vi "test.OutputStream.vi"(8 "error in":errorcluster, 10 "Data":variant, 11 "Command":string) -> (0 "error out":errorcluster, 3 "Return Data":variant)   [LabVIEW 2014]
uses:
  Private/Class/meth.Constructor.vi
  Private/Class/meth.SetStreamReader.vi
  Private/Class/meth.Destructor.vi
  Private/Class/meth.ExecFunction.vi
  GLue.lvlib
panel:
  out "String":string
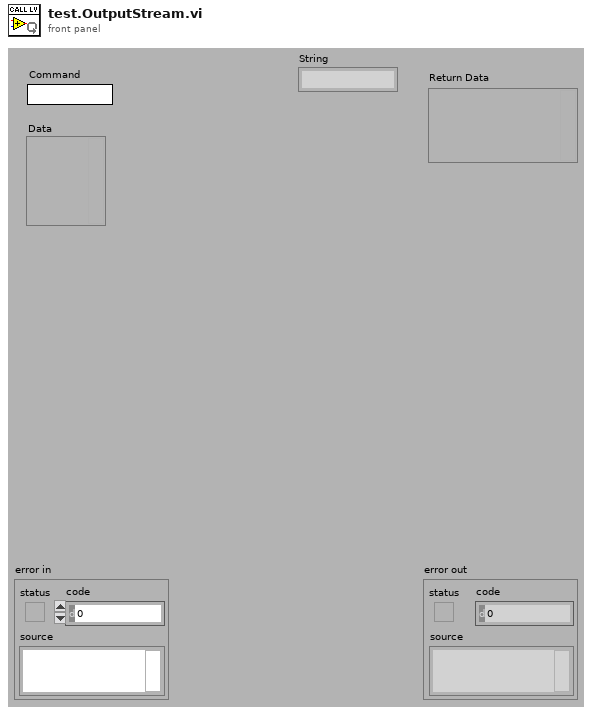
[diagram p1: front panel]
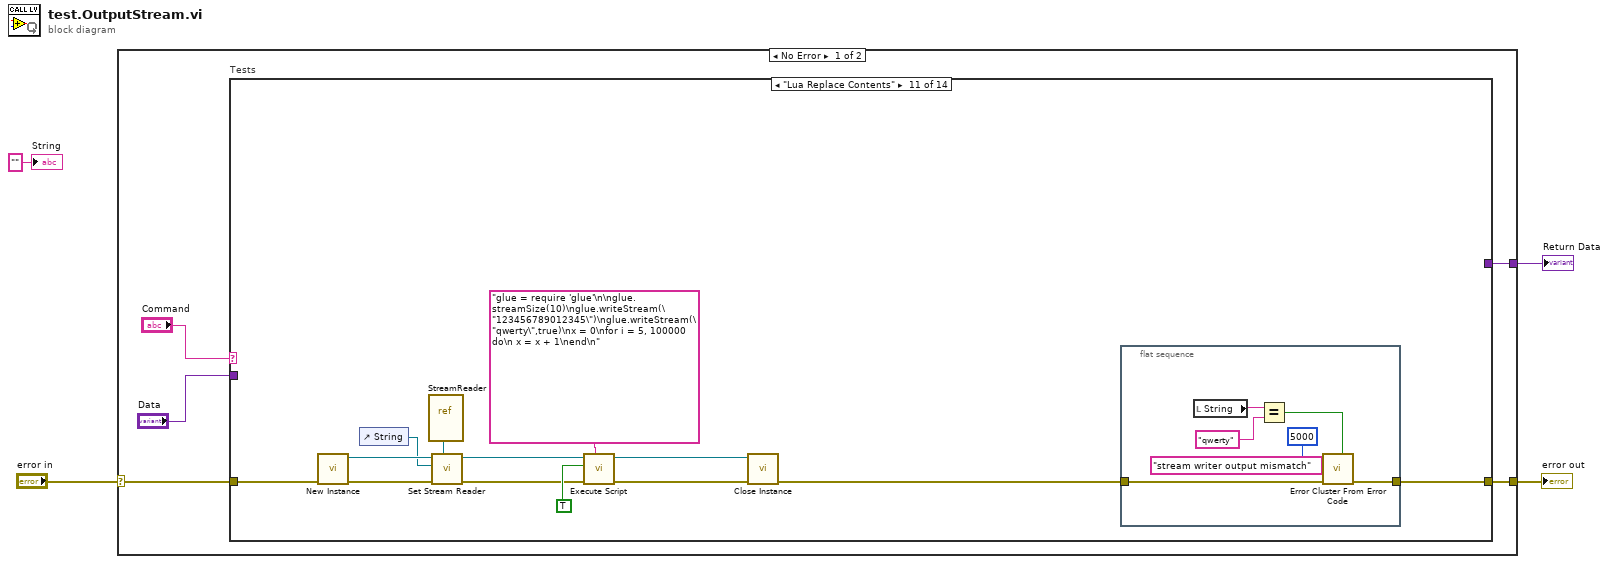
[diagram p0: block diagram]
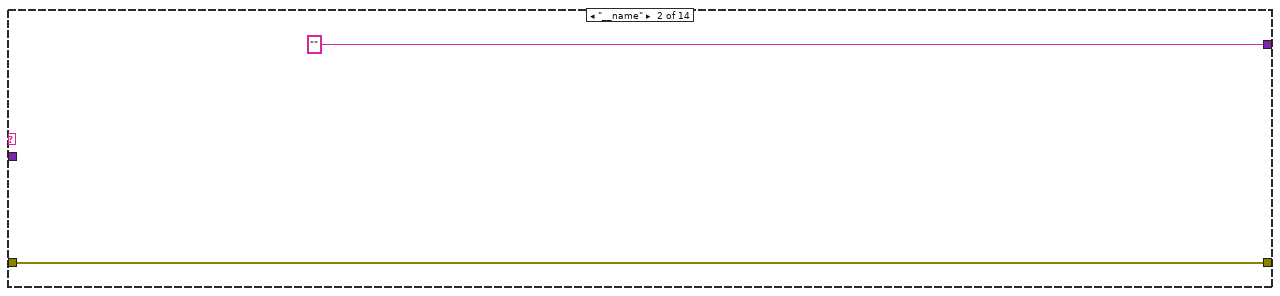
[diagram p3: hidden frame]
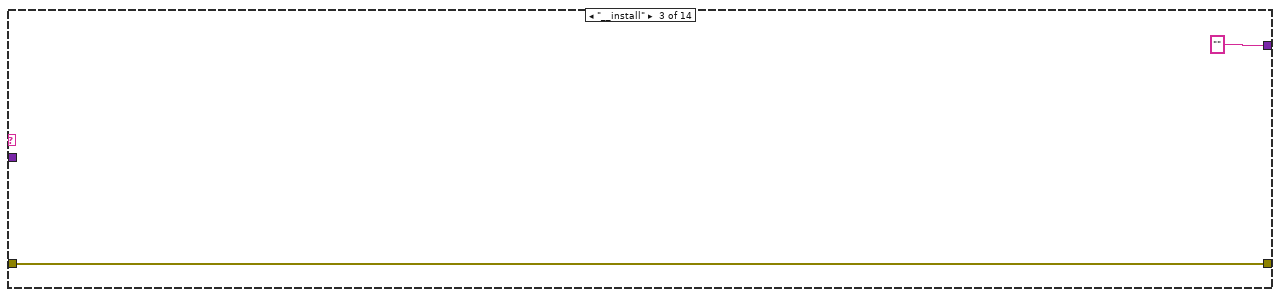
[diagram p4: hidden frame]
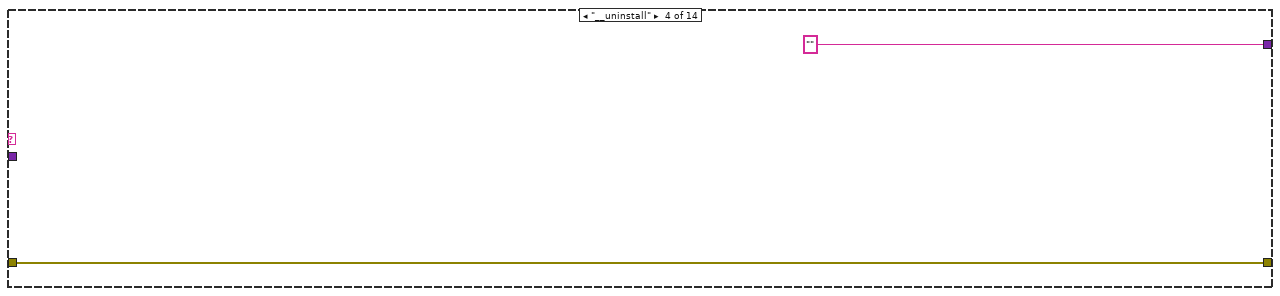
[diagram p5: hidden frame]
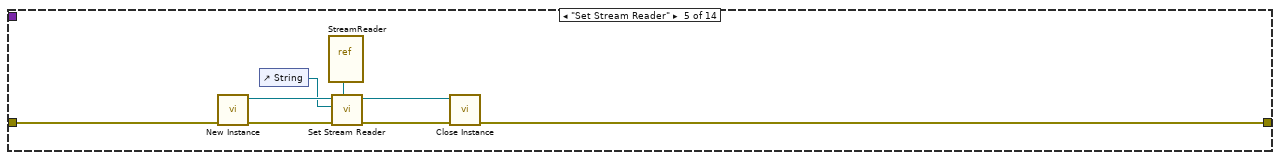
[diagram p6: hidden frame]
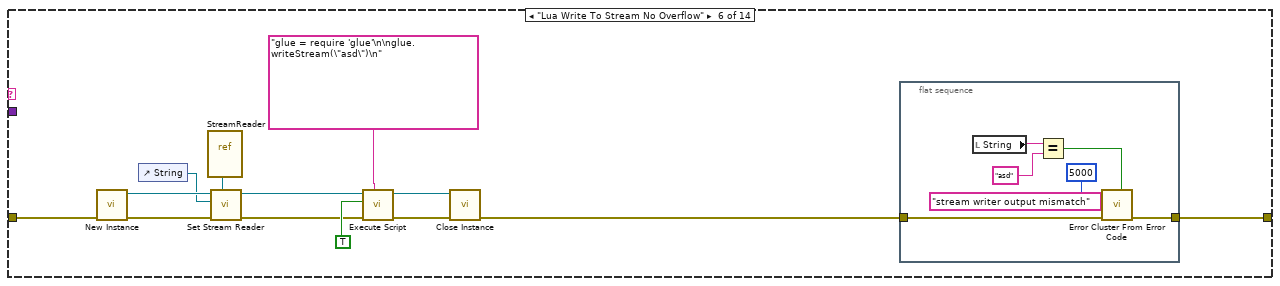
[diagram p7: hidden frame]
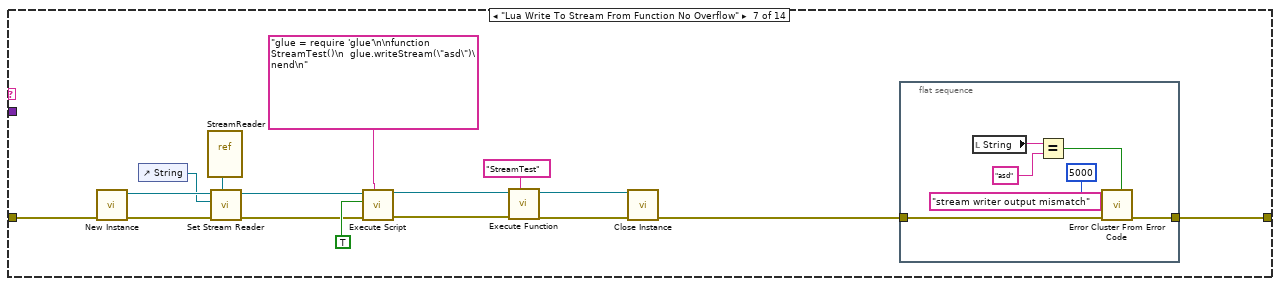
[diagram p8: hidden frame]
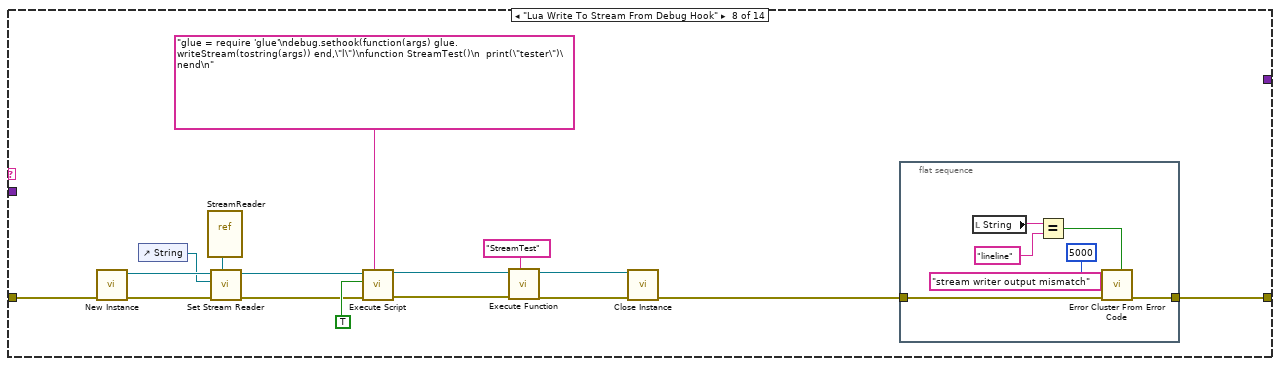
[diagram p9: hidden frame]
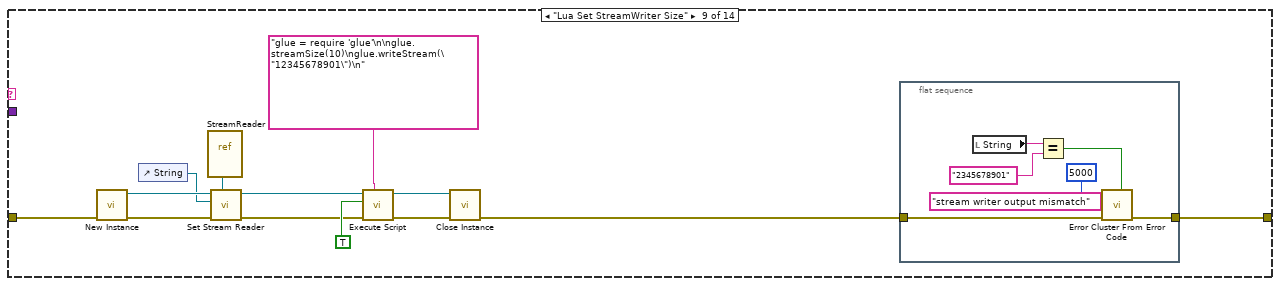
[diagram p10: hidden frame]
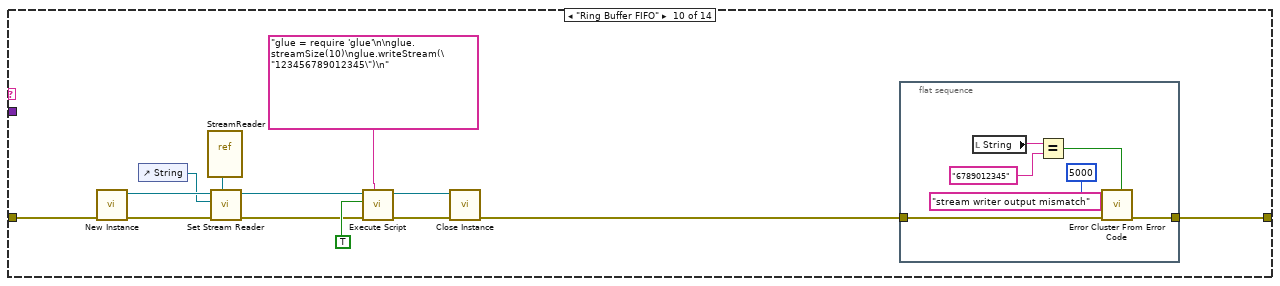
[diagram p11: hidden frame]
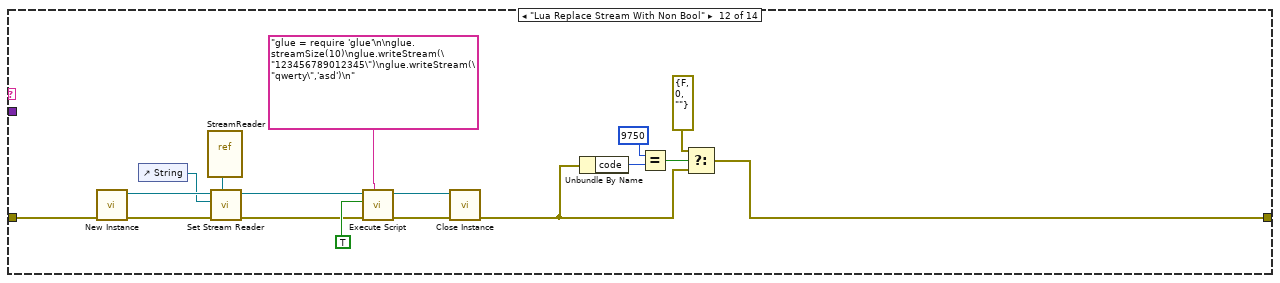
[diagram p12: hidden frame]
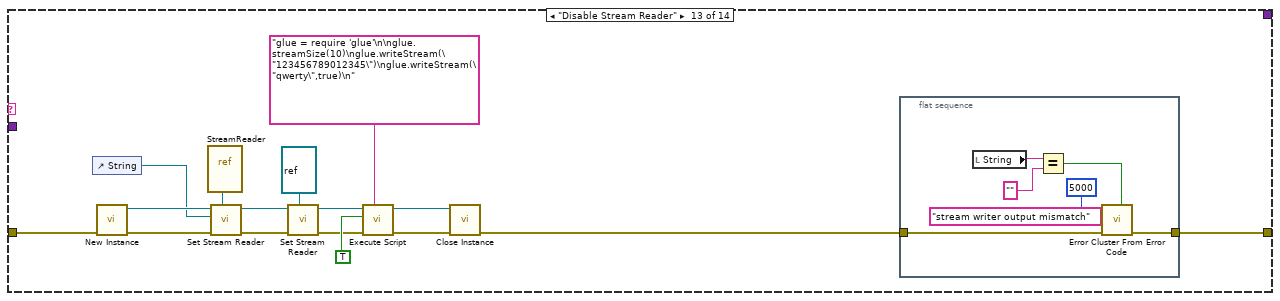
[diagram p13: hidden frame]
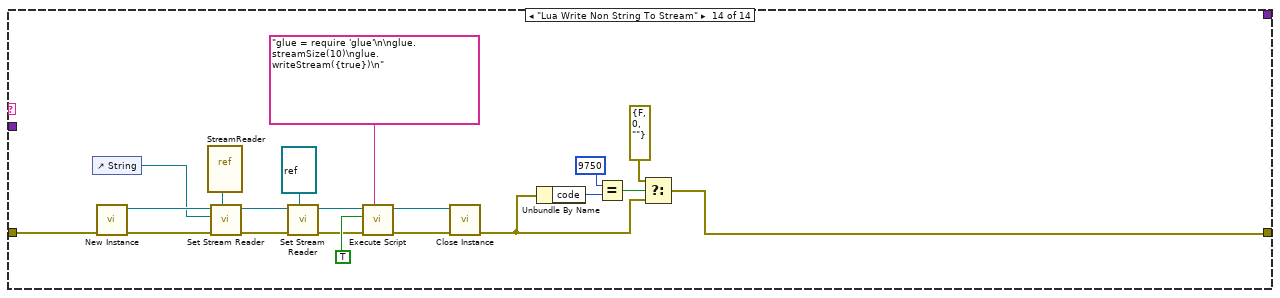
[diagram p14: hidden frame]
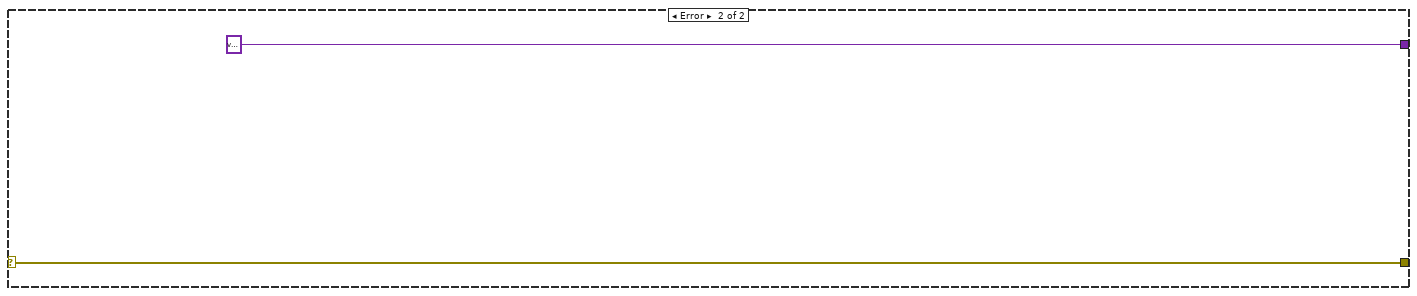
[diagram p15: hidden frame]
diagram:
  n1 = case shown="No Error" "error in" {
    selector: "error in" -> [w9 w213]
    tunnel: [w7 w213] -> w3
    tunnel: [w8 variant ("User Data")] -> w2
    frame No Error {
      n2 = case "Tests" shown="\"Lua Replace Contents\"" "Command" {
        tunnel: w9 -> [w11 w12 w14 w16 w25 w38 w61 w84 w104 w124 w144 w168 w184 w211]
        tunnel: "Data" -> [w10 _ _ _ _ _ _ _ _ _ _ _ _ _]
        tunnel: [w10 "" "" "" _ _ _ _ _ _ _ _ _ _] -> w8
        tunnel: [w11 w12 w14 w16 w24 w26 w51 w74 w92 w112 w132 w152 w174 w192] -> w7
        frame Default {
        }
        frame "__name" {
        }
        frame "__install" {
        }
        frame "__uninstall" {
        }
        frame "Set Stream Reader" {
          n3 = call "New Instance.vi"("error in"=w25) -> ("error out"=w23:errorcluster, "GLue out"=w22:refnum<class "class.GLue.lvclass">)  [unwired: 9 in]
          n4 = control-ref of="String"() -> (w20:refnum<vi>)
          n5 = vi-ref "StreamReader.vi"() -> (w21:refnum<vi>)
          n6 = call "Set Stream Reader.vi"("StreamReader"=w21, "error in"=w23, "UserData"=w20, "GLue in"=w22) -> ("error out"=w19:errorcluster, "GLue out"=w18:refnum<class "class.GLue.lvclass">)  [unwired: 6 in]
          n7 = call "Close Instance.vi"("error in"=w19, "GLue in"=w18) -> ("error out"=w24:errorcluster)  [unwired: 9 in]
        }
        frame "Lua Write To Stream No Overflow" {
          n8 = call "New Instance.vi"("error in"=w38) -> ("error out"=w33:errorcluster, "GLue out"=w30:refnum<class "class.GLue.lvclass">)  [unwired: 9 in]
          n9 = control-ref of="String"() -> (w28:refnum<vi>)
          n10 = vi-ref "StreamReader.vi"() -> (w29:refnum<vi>)
          n11 = call "Set Stream Reader.vi"("StreamReader"=w29, "error in"=w33, "UserData"=w28, "GLue in"=w30) -> ("error out"=w32:errorcluster, "GLue out"=w31:refnum<class "class.GLue.lvclass">)  [unwired: 6 in]
          n12 = call "Execute Script.vi"("Script"="glue = require 'glue'\n\nglue.writeStream(\"asd\")\n", "error in"=w32, "Argument Data"=TRUE, "GLue in"=w31) -> ("error out"=w35:errorcluster, "GLue out"=w34:refnum<class "class.GLue.lvclass">)  [unwired: 5 in, 1 out]
          n13 = call "Close Instance.vi"("error in"=w35, "GLue in"=w34) -> ("error out"=w27:errorcluster)  [unwired: 9 in]
          n14 = flat-sequence {
            tunnel: w27 -> [w43]
            tunnel: [w42] -> w26
            frame #0 {
              n15 = local read "String"() -> (w45:string)
              n16 = Equal?(x=w45, y="asd") -> (x = y?=w41:bool)
              n17 = call <vilib>:"Error Cluster From Error Code.vi"("is warning? (False)"=w41, "error in (no error)"=w43, "error message (\"\")"="stream writer output mismatch" ("error message (\"\")"), "error code (0)"=5000) -> ("error out"=w42:errorcluster)  [unwired: 5 in]
            }
          }
        }
        frame "Lua Write To Stream From Function No Overflow" {
          n18 = call "New Instance.vi"("error in"=w61) -> ("error out"=w58:errorcluster, "GLue out"=w55:refnum<class "class.GLue.lvclass">)  [unwired: 9 in]
          n19 = control-ref of="String"() -> (w53:refnum<vi>)
          n20 = vi-ref "StreamReader.vi"() -> (w54:refnum<vi>)
          n21 = call "Set Stream Reader.vi"("StreamReader"=w54, "error in"=w58, "UserData"=w53, "GLue in"=w55) -> ("error out"=w57:errorcluster, "GLue out"=w56:refnum<class "class.GLue.lvclass">)  [unwired: 6 in]
          n22 = call "Execute Script.vi"("Script"="glue = require 'glue'\n\nfunction StreamTest()\n  glue.writeStream(\"asd\")\nend\n", "error in"=w57, "Argument Data"=TRUE, "GLue in"=w56) -> ("error out"=w50:errorcluster, "GLue out"=w49:refnum<class "class.GLue.lvclass">)  [unwired: 5 in, 1 out]
          n23 = call "Execute Function.vi"("Function Name"="StreamTest", "error in"=w50, "GLue in"=w49) -> ("error out"=w47:errorcluster, "GLue out"=w48:refnum<class "class.GLue.lvclass">)  [unwired: 6 in, 1 out]
          n24 = call "Close Instance.vi"("error in"=w47, "GLue in"=w48) -> ("error out"=w52:errorcluster)  [unwired: 9 in]
          n25 = flat-sequence {
            tunnel: w52 -> [w66]
            tunnel: [w65] -> w51
            frame #0 {
              n26 = local read "String"() -> (w68:string)
              n27 = Equal?(x=w68, y="asd") -> (x = y?=w64:bool)
              n28 = call <vilib>:"Error Cluster From Error Code.vi"("is warning? (False)"=w64, "error in (no error)"=w66, "error message (\"\")"="stream writer output mismatch" ("error message (\"\")"), "error code (0)"=5000) -> ("error out"=w65:errorcluster)  [unwired: 5 in]
            }
          }
        }
        frame "Lua Write To Stream From Debug Hook" {
          n29 = call "New Instance.vi"("error in"=w84) -> ("error out"=w81:errorcluster, "GLue out"=w78:refnum<class "class.GLue.lvclass">)  [unwired: 9 in]
          n30 = control-ref of="String"() -> (w76:refnum<vi>)
          n31 = vi-ref "StreamReader.vi"() -> (w77:refnum<vi>)
          n32 = call "Set Stream Reader.vi"("StreamReader"=w77, "error in"=w81, "UserData"=w76, "GLue in"=w78) -> ("error out"=w80:errorcluster, "GLue out"=w79:refnum<class "class.GLue.lvclass">)  [unwired: 6 in]
          n33 = call "Execute Script.vi"("Script"="glue = require 'glue'\ndebug.sethook(function(args) glue.writeStream(tostring(args)) end,\"l\")\nfunction StreamTest()\n  print(\"tester\")\nend\n", "error in"=w80, "Argument Data"=TRUE, "GLue in"=w79) -> ("error out"=w73:errorcluster, "GLue out"=w72:refnum<class "class.GLue.lvclass">)  [unwired: 5 in, 1 out]
          n34 = call "Execute Function.vi"("Function Name"="StreamTest", "error in"=w73, "GLue in"=w72) -> ("error out"=w70:errorcluster, "GLue out"=w71:refnum<class "class.GLue.lvclass">)  [unwired: 6 in, 1 out]
          n35 = call "Close Instance.vi"("error in"=w70, "GLue in"=w71) -> ("error out"=w75:errorcluster)  [unwired: 9 in]
          n36 = flat-sequence {
            tunnel: w75 -> [w89]
            tunnel: [w88] -> w74
            frame #0 {
              n37 = local read "String"() -> (w91:string)
              n38 = Equal?(x=w91, y="lineline") -> (x = y?=w87:bool)
              n39 = call <vilib>:"Error Cluster From Error Code.vi"("is warning? (False)"=w87, "error in (no error)"=w89, "error message (\"\")"="stream writer output mismatch" ("error message (\"\")"), "error code (0)"=5000) -> ("error out"=w88:errorcluster)  [unwired: 5 in]
            }
          }
        }
        frame "Lua Set StreamWriter Size" {
          n40 = call "New Instance.vi"("error in"=w104) -> ("error out"=w99:errorcluster, "GLue out"=w96:refnum<class "class.GLue.lvclass">)  [unwired: 9 in]
          n41 = control-ref of="String"() -> (w94:refnum<vi>)
          n42 = vi-ref "StreamReader.vi"() -> (w95:refnum<vi>)
          n43 = call "Set Stream Reader.vi"("StreamReader"=w95, "error in"=w99, "UserData"=w94, "GLue in"=w96) -> ("error out"=w98:errorcluster, "GLue out"=w97:refnum<class "class.GLue.lvclass">)  [unwired: 6 in]
          n44 = call "Execute Script.vi"("Script"="glue = require 'glue'\n\nglue.streamSize(10)\nglue.writeStream(\"12345678901\")\n", "error in"=w98, "Argument Data"=TRUE, "GLue in"=w97) -> ("error out"=w101:errorcluster, "GLue out"=w100:refnum<class "class.GLue.lvclass">)  [unwired: 5 in, 1 out]
          n45 = call "Close Instance.vi"("error in"=w101, "GLue in"=w100) -> ("error out"=w93:errorcluster)  [unwired: 9 in]
          n46 = flat-sequence {
            tunnel: w93 -> [w109]
            tunnel: [w108] -> w92
            frame #0 {
              n47 = local read "String"() -> (w111:string)
              n48 = Equal?(x=w111, y="2345678901") -> (x = y?=w107:bool)
              n49 = call <vilib>:"Error Cluster From Error Code.vi"("is warning? (False)"=w107, "error in (no error)"=w109, "error message (\"\")"="stream writer output mismatch" ("error message (\"\")"), "error code (0)"=5000) -> ("error out"=w108:errorcluster)  [unwired: 5 in]
            }
          }
        }
        frame "Ring Buffer FIFO" {
          n50 = call "New Instance.vi"("error in"=w124) -> ("error out"=w119:errorcluster, "GLue out"=w116:refnum<class "class.GLue.lvclass">)  [unwired: 9 in]
          n51 = control-ref of="String"() -> (w114:refnum<vi>)
          n52 = vi-ref "StreamReader.vi"() -> (w115:refnum<vi>)
          n53 = call "Set Stream Reader.vi"("StreamReader"=w115, "error in"=w119, "UserData"=w114, "GLue in"=w116) -> ("error out"=w118:errorcluster, "GLue out"=w117:refnum<class "class.GLue.lvclass">)  [unwired: 6 in]
          n54 = call "Execute Script.vi"("Script"="glue = require 'glue'\n\nglue.streamSize(10)\nglue.writeStream(\"123456789012345\")\n", "error in"=w118, "Argument Data"=TRUE, "GLue in"=w117) -> ("error out"=w121:errorcluster, "GLue out"=w120:refnum<class "class.GLue.lvclass">)  [unwired: 5 in, 1 out]
          n55 = call "Close Instance.vi"("error in"=w121, "GLue in"=w120) -> ("error out"=w113:errorcluster)  [unwired: 9 in]
          n56 = flat-sequence {
            tunnel: w113 -> [w129]
            tunnel: [w128] -> w112
            frame #0 {
              n57 = local read "String"() -> (w131:string)
              n58 = Equal?(x=w131, y="6789012345") -> (x = y?=w127:bool)
              n59 = call <vilib>:"Error Cluster From Error Code.vi"("is warning? (False)"=w127, "error in (no error)"=w129, "error message (\"\")"="stream writer output mismatch" ("error message (\"\")"), "error code (0)"=5000) -> ("error out"=w128:errorcluster)  [unwired: 5 in]
            }
          }
        }
        frame "Lua Replace Contents" {
          n60 = call "New Instance.vi"("error in"=w144) -> ("error out"=w139:errorcluster, "GLue out"=w136:refnum<class "class.GLue.lvclass">)  [unwired: 9 in]
          n61 = control-ref of="String"() -> (w134:refnum<vi>)
          n62 = vi-ref "StreamReader.vi"() -> (w135:refnum<vi>)
          n63 = call "Set Stream Reader.vi"("StreamReader"=w135, "error in"=w139, "UserData"=w134, "GLue in"=w136) -> ("error out"=w138:errorcluster, "GLue out"=w137:refnum<class "class.GLue.lvclass">)  [unwired: 6 in]
          n64 = call "Execute Script.vi"("Script"="glue = require 'glue'\n\nglue.streamSize(10)\nglue.writeStream(\"123456789012345\")\nglue.writeStream(\"qwerty\",true)\nx = 0\nfor i = 5, 100000 do\n x = x + 1\nend\n", "error in"=w138, "Argument Data"=TRUE, "GLue in"=w137) -> ("error out"=w141:errorcluster, "GLue out"=w140:refnum<class "class.GLue.lvclass">)  [unwired: 5 in, 1 out]
          n65 = call "Close Instance.vi"("error in"=w141, "GLue in"=w140) -> ("error out"=w133:errorcluster)  [unwired: 9 in]
          n66 = flat-sequence {
            tunnel: w133 -> [w149]
            tunnel: [w148] -> w132
            frame #0 {
              n67 = local read "String"() -> (w151:string)
              n68 = Equal?(x=w151, y="qwerty") -> (x = y?=w147:bool)
              n69 = call <vilib>:"Error Cluster From Error Code.vi"("is warning? (False)"=w147, "error in (no error)"=w149, "error message (\"\")"="stream writer output mismatch" ("error message (\"\")"), "error code (0)"=5000) -> ("error out"=w148:errorcluster)  [unwired: 5 in]
            }
          }
        }
        frame "Lua Replace Stream With Non Bool" {
          n70 = call "New Instance.vi"("error in"=w168) -> ("error out"=w163:errorcluster, "GLue out"=w160:refnum<class "class.GLue.lvclass">)  [unwired: 9 in]
          n71 = control-ref of="String"() -> (w158:refnum<vi>)
          n72 = vi-ref "StreamReader.vi"() -> (w159:refnum<vi>)
          n73 = call "Set Stream Reader.vi"("StreamReader"=w159, "error in"=w163, "UserData"=w158, "GLue in"=w160) -> ("error out"=w162:errorcluster, "GLue out"=w161:refnum<class "class.GLue.lvclass">)  [unwired: 6 in]
          n74 = call "Execute Script.vi"("Script"="glue = require 'glue'\n\nglue.streamSize(10)\nglue.writeStream(\"123456789012345\")\nglue.writeStream(\"qwerty\",'asd')\n", "error in"=w162, "Argument Data"=TRUE, "GLue in"=w161) -> ("error out"=w165:errorcluster, "GLue out"=w164:refnum<class "class.GLue.lvclass">)  [unwired: 5 in, 1 out]
          n75 = call "Close Instance.vi"("error in"=w165, "GLue in"=w164) -> ("error out"=w153:errorcluster)  [unwired: 9 in]
          n76 = Unbundle By Name(w153) -> ("code"=w156:i32)
          n77 = Equal?(x=9750, y=w156) -> (x = y?=w155:bool)
          n78 = Select(t=errorcluster {"status"=FALSE, "code"=0, "source"=""} ("error out"), s=w155, f=w153) -> (s? t:f=w152:errorcluster)
        }
        frame "Disable Stream Reader" {
          n79 = control-ref of="String"() -> (w176:refnum<vi>)
          n80 = call "New Instance.vi"("error in"=w184) -> ("error out"=w179:errorcluster, "GLue out"=w178:refnum<class "class.GLue.lvclass">)  [unwired: 9 in]
          n81 = vi-ref "StreamReader.vi"() -> (w177:refnum<vi>)
          n82 = call "Set Stream Reader.vi"("StreamReader"=w177, "error in"=w179, "UserData"=w176, "GLue in"=w178) -> ("error out"=w173:errorcluster, "GLue out"=w172:refnum<class "class.GLue.lvclass">)  [unwired: 6 in]
          n83 = call "Set Stream Reader.vi"("StreamReader"=refnum<vi> refnum, "error in"=w173, "GLue in"=w172) -> ("error out"=w170:errorcluster, "GLue out"=w171:refnum<class "class.GLue.lvclass">)  [unwired: 7 in]
          n84 = call "Execute Script.vi"("Script"="glue = require 'glue'\n\nglue.streamSize(10)\nglue.writeStream(\"123456789012345\")\nglue.writeStream(\"qwerty\",true)\n", "error in"=w170, "Argument Data"=TRUE, "GLue in"=w171) -> ("error out"=w181:errorcluster, "GLue out"=w180:refnum<class "class.GLue.lvclass">)  [unwired: 5 in, 1 out]
          n85 = call "Close Instance.vi"("error in"=w181, "GLue in"=w180) -> ("error out"=w175:errorcluster)  [unwired: 9 in]
          n86 = flat-sequence {
            tunnel: w175 -> [w189]
            tunnel: [w188] -> w174
            frame #0 {
              n87 = local read "String"() -> (w191:string)
              n88 = Equal?(x=w191, y="") -> (x = y?=w187:bool)
              n89 = call <vilib>:"Error Cluster From Error Code.vi"("is warning? (False)"=w187, "error in (no error)"=w189, "error message (\"\")"="stream writer output mismatch" ("error message (\"\")"), "error code (0)"=5000) -> ("error out"=w188:errorcluster)  [unwired: 5 in]
            }
          }
        }
        frame "Lua Write Non String To Stream" {
          n90 = control-ref of="String"() -> (w203:refnum<vi>)
          n91 = call "New Instance.vi"("error in"=w211) -> ("error out"=w206:errorcluster, "GLue out"=w205:refnum<class "class.GLue.lvclass">)  [unwired: 9 in]
          n92 = vi-ref "StreamReader.vi"() -> (w204:refnum<vi>)
          n93 = call "Set Stream Reader.vi"("StreamReader"=w204, "error in"=w206, "UserData"=w203, "GLue in"=w205) -> ("error out"=w202:errorcluster, "GLue out"=w201:refnum<class "class.GLue.lvclass">)  [unwired: 6 in]
          n94 = call "Set Stream Reader.vi"("StreamReader"=refnum<vi> refnum, "error in"=w202, "GLue in"=w201) -> ("error out"=w199:errorcluster, "GLue out"=w200:refnum<class "class.GLue.lvclass">)  [unwired: 7 in]
          n95 = call "Execute Script.vi"("Script"="glue = require 'glue'\n\nglue.streamSize(10)\nglue.writeStream({true})\n", "error in"=w199, "Argument Data"=TRUE, "GLue in"=w200) -> ("error out"=w208:errorcluster, "GLue out"=w207:refnum<class "class.GLue.lvclass">)  [unwired: 5 in, 1 out]
          n96 = call "Close Instance.vi"("error in"=w208, "GLue in"=w207) -> ("error out"=w193:errorcluster)  [unwired: 9 in]
          n97 = Unbundle By Name(w193) -> ("code"=w196:i32)
          n98 = Equal?(x=9750, y=w196) -> (x = y?=w195:bool)
          n99 = Select(t=errorcluster {"status"=FALSE, "code"=0, "source"=""} ("error out"), s=w195, f=w193) -> (s? t:f=w192:errorcluster)
        }
      }
    }
    frame Error {
    }
  }
  "Return Data" <- w2
  "error out" <- w3
  "String" <- "" ("String")
